vi "ClientDaemon.vi"(8 "error in (no error)":errorcluster, 10 "MessageReceiveQueue":refnum<queue>, 11 "mqtt.lvclass":refnum<class "MQTT Client.lvclass">) -> (0 "error out":errorcluster, 3 "mqtt.lvclass 2":refnum<class "MQTT Client.lvclass">)   [LabVIEW 2020, in "MQTT Client.lvclass"]
uses:
  MQTT Client.lvclass
  MqttMessage.ctl
  MQTT Client.lvclass/MQTT Client.ctl
  mqttTypedef/ReceivedData.ctl
  mqttTypedef/FixedHeaderResponse.ctl
  mqttTypedef/QosLevel.ctl
  mqttTypedef/MessageType.ctl
  mqttCmd/mqttCmdPublishAck/PublishAckMqttMsg.lvclass
  C:/Projects/Libraries/Gore SM 2020/mqtt-LabVIEW/src/class/mqtt/mqttCmd/BaseMqttMsg.lvclass
  mqttCmd/mqttCmdPublishReceived/PublishReceivedMqttMsg.lvclass
  mqttCmd/mqttCmdPublishComplete/PublishCompleteMqttMsg.lvclass
  mqttCmd/mqttCmdPingResponse/PingResponseMqttMsg.lvclass
  mqttCmd/BaseMqttMsg.lvclass
panel:
  out "rxCount":i32
  out "rxTelegram":u8[](array[numeric]) format="%02x"
  out "txError":errorcluster
  out "payloadError":errorcluster
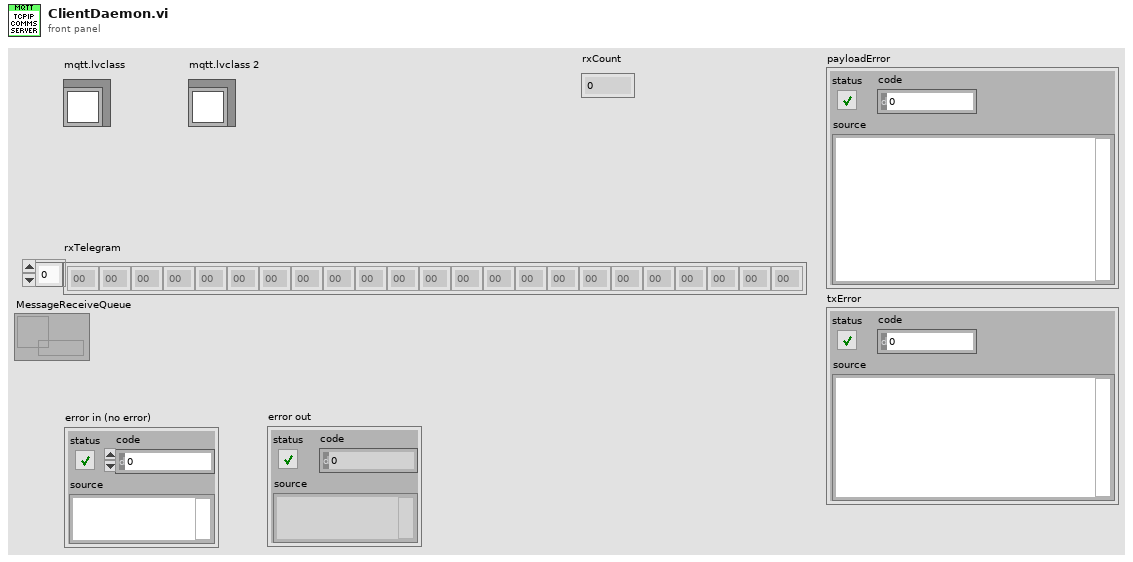
[diagram p1: front panel]
types:
  T1 = typedef "MQTT Client.lvclass/ReceivedData.ctl" = cluster{"fixedHdr":T2, "payload":u8[]}
  T2 = typedef "MQTT Client.lvclass/FixedHeaderResponse.ctl" = cluster{"retain":bool, "qos":T3, "duplicate":bool, "response":T4}
  T3 = typedef "MQTT Client.lvclass/QosLevel.ctl" = enum8{"At most once", "At least once", "Exactly once", "Reserved"}
  T4 = typedef "MQTT Client.lvclass/MessageType.ctl" = enum32{"Reserved", "CONNECT", "CONNACK", "PUBLISH", "PUBACK", "PUBREC", "PUBREL", "PUBCOMP", "SUBSCRIBE", "SUBACK", "UNSUBSCRIBE", "UNSUBACK", "PINGREQ", "PINGRESP", "DISCONNECT", "Reserved2"}
  T5 = cluster{"topic":string, "value":string, "messageID":u16}
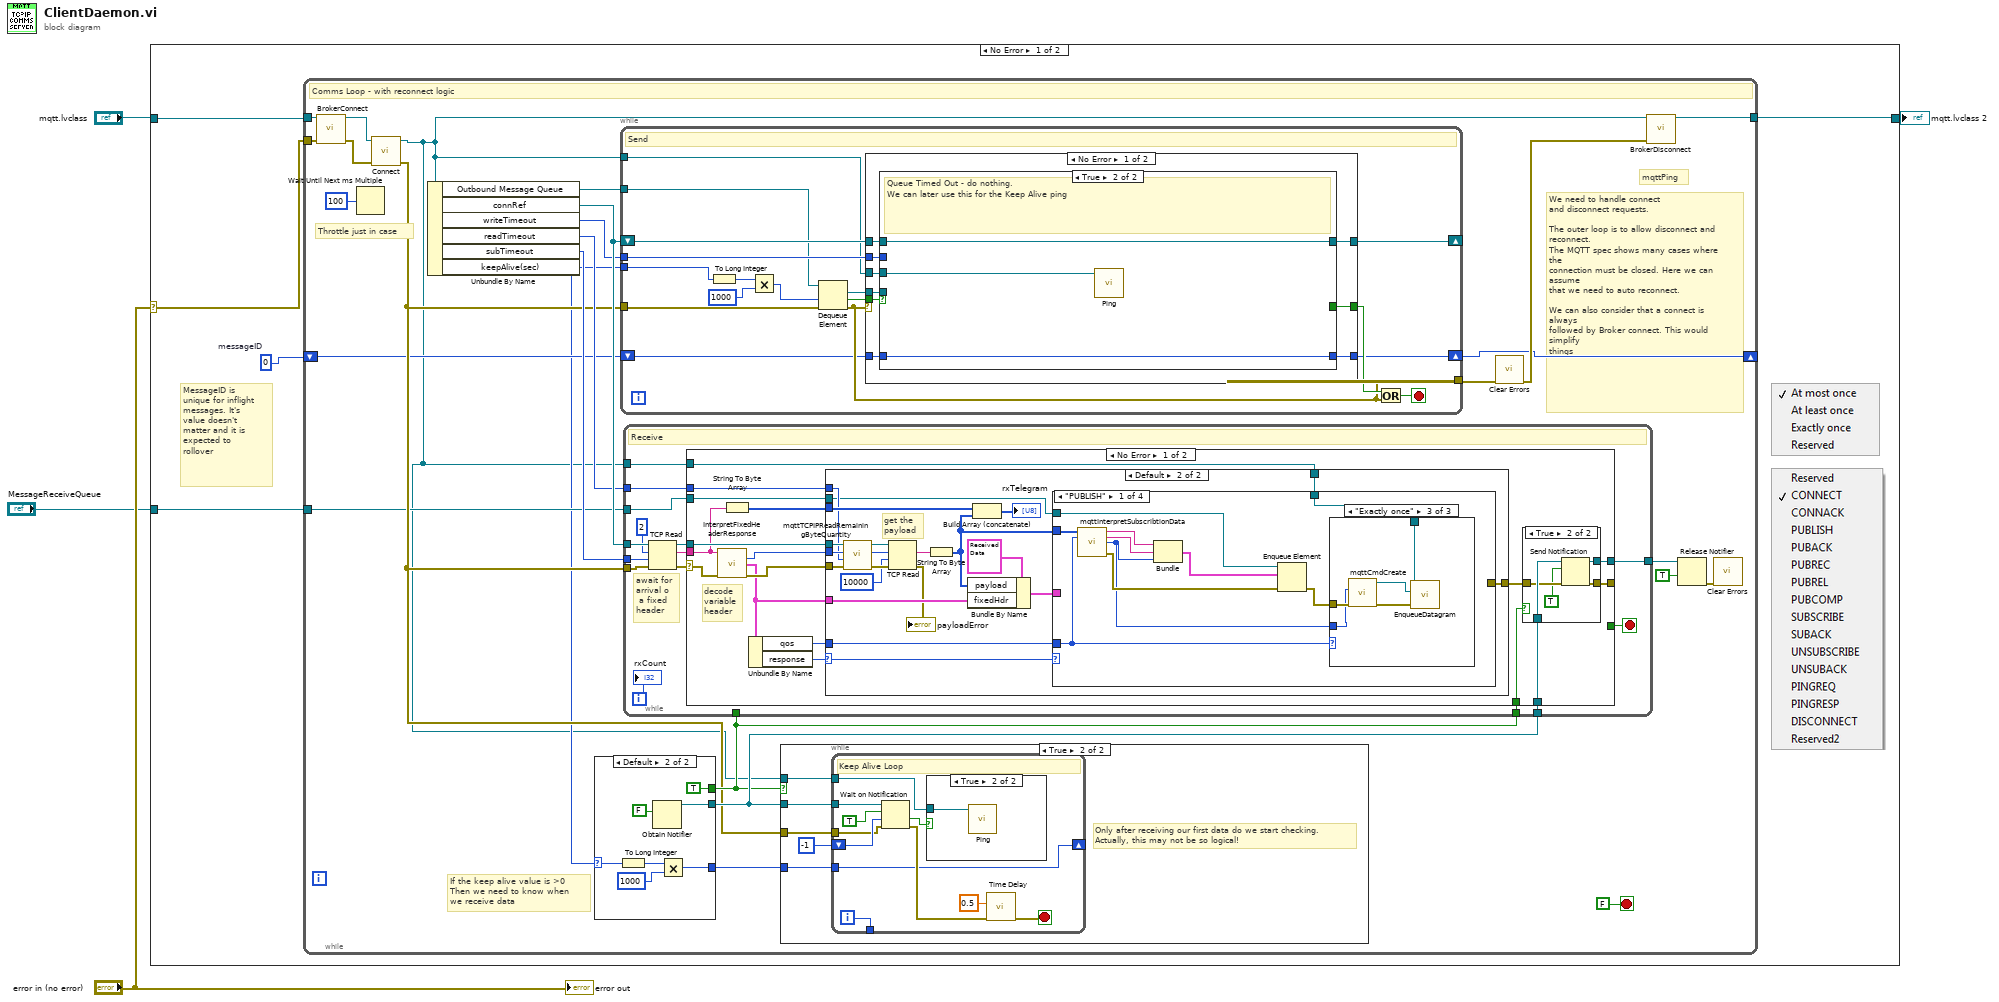
[diagram p0: block diagram]
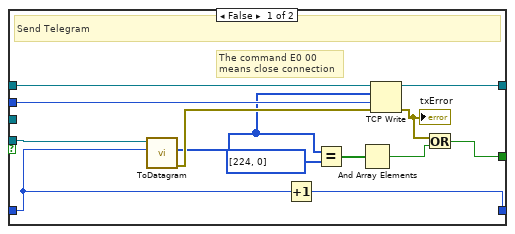
[diagram p5: hidden frame]
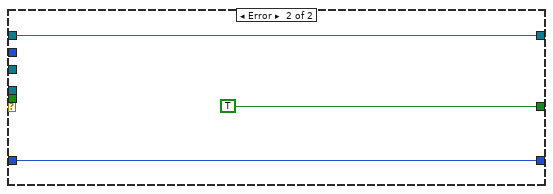
[diagram p6: hidden frame]
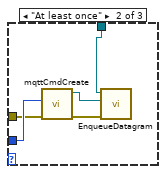
[diagram p10: hidden frame]
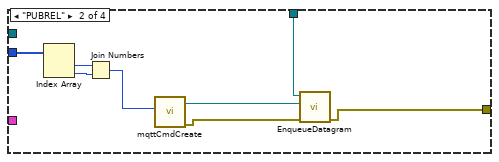
[diagram p11: hidden frame]
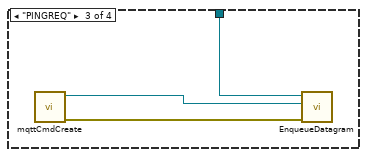
[diagram p12: hidden frame]
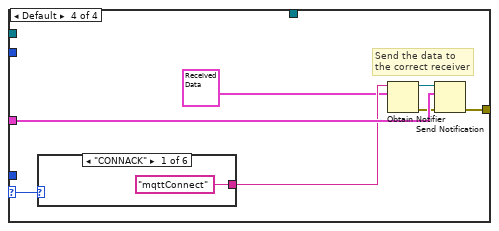
[diagram p13: hidden frame]
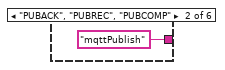
[diagram p14: hidden frame]
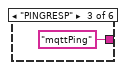
[diagram p15: hidden frame]
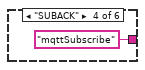
[diagram p16: hidden frame]
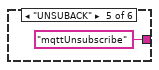
[diagram p17: hidden frame]
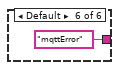
[diagram p18: hidden frame]
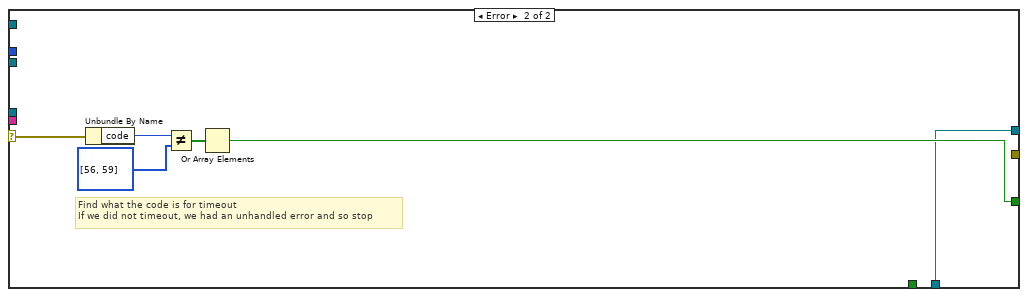
[diagram p19: hidden frame]
diagram:
  n1 = case shown="No Error" "error in (no error)" {
    selector: "error in (no error)" -> [w8 _]
    tunnel: "mqtt.lvclass" -> [w6 w213]
    tunnel: [w9 w213] -> w3
    tunnel: "MessageReceiveQueue" -> [w7 _]
    frame No Error {
      w5 = u16 0  # messageID
      # "MessageID is unique for inflight messages. It's value doesn't matter and it is expected to rollover"
      n2 = while {
        tunnel: w6 -> [w31]
        tunnel: [w29] -> w9
        tunnel: w8 -> [w30]
        tunnel: w7 -> [w17]
        shift-right: [w12] -> _
        shift-left: w5 -> [w13]
        stop <- FALSE stop-if-true
        # "We need to handle connect\nand disconnect requests.\n\nThe outer loop is to allow disconnect and reconnect.\nThe MQTT spec shows many cases where the\nconnection must be closed. Here we can assume\nthat we need to auto reconnect.\n\nWe can also consider that a connect is always\nfollowed by Broker connect. This would simplify\nthings"
        # "Throttle just in case"
        # "If the keep alive value is >0\nThen we need to know when\nwe receive data"
        # "mqttPing"
        # "Comms Loop - with reconnect logic"
        n3 = call "BrokerConnect.vi"("mqtt in"=w31, "error in (no error)"=w30) -> ("mqtt out"=w15:refnum<class "MQTT Client.lvclass">, "error out"=w19:errorcluster)  [unwired: 12 in]
        n4 = Wait Until Next ms Multiple(millisecond multiple=u32 100) -> ()  [unwired: 1 out]
        n5 = call "Connect.vi"("error in (no error)"=w19, "MQTT In"=w15) -> ("error out"=w18:errorcluster, "MQTT Out"=w10:refnum<class "MQTT Client.lvclass">)  [unwired: 8 in]
        n6 = Unbundle By Name(w10) -> ("Outbound Message Queue"=w14:refnum<queue>, "connRef"=w34:refnum<k5>, "writeTimeout"=w28:i32, "readTimeout"=w27:i32, "subTimeout"=w26:i32, "keepAlive(sec)"=w11:u16)
        n7 = case shown="Default" w11 {
          selector: w11 -> [_ w54]
          tunnel: [_ w59] -> w25
          tunnel: [_ w55] -> w21
          tunnel: [_ TRUE] -> w20
          frame ..0 {
          }
          frame Default {
            n8 = To Long Integer(number=w54) -> (32bit integer=w57:i32)
            n9 = Obtain Notifier(notification data type=FALSE) -> (notifier out=w59:refnum<notifier>)  [unwired: 3 in, 2 out]
            n10 = Multiply(x=w57, y=1000) -> (x*y=w55:i32)
          }
        }
        n11 = while {
          shift-right: [w74] -> _
          shift-left: w34 -> [w75]
          tunnel: [w70] -> w33
          tunnel: w28 -> [w69]
          tunnel: w18 -> [w68]
          tunnel: w14 -> [w67]
          shift-right: [w65] -> w12
          shift-left: w13 -> [w66]
          tunnel: w11 -> [w62]
          tunnel: w10 -> [w60]
          stop <- w73 stop-if-true
          # "Send"
          n12 = To Long Integer(number=w62) -> (32bit integer=w63:i32)
          n13 = Multiply(x=w63, y=1000) -> (x*y=w61:i32)
          n14 = Dequeue Element(queue=w67, timeout in ms (-1)=w61, error in (no error)=w68) -> (element=w71:refnum<class "BaseMqttMsg.lvclass">, timed out?=w76:bool, error out=w70:errorcluster)  [unwired: 1 out]
          n15 = case shown="No Error" w70 {
            tunnel: w76 -> [w85 _]
            tunnel: w71 -> [w84 _]
            tunnel: w75 -> [w83 w104]
            tunnel: [w82 w104] -> w74
            tunnel: [w81 TRUE] -> w72
            tunnel: w69 -> [w80 _]
            tunnel: w66 -> [w79 w102]
            tunnel: [w78 w102] -> w65
            tunnel: w60 -> [w77 _]
            frame No Error {
              n16 = case shown="True" w85 {
                tunnel: w84 -> [w90 _]
                tunnel: w83 -> [w98 w101]
                tunnel: [w97 w101] -> w82
                tunnel: [w91 _] -> w81
                tunnel: w80 -> [w94 _]
                tunnel: w79 -> [w87 w100]
                tunnel: [w86 w100] -> w78
                tunnel: w77 -> [_ w99]
                frame False {
                  # "The command E0 00\nmeans close connection"
                  # "Send Telegram"
                  n17 = call-dynamic "ToDatagram.vi"("messageID"=w87, "BaseMqttMsg in"=w90) -> ("error out"=w89:errorcluster, "Datagram"=w88:u8[])  [unwired: 7 in, 1 out]
                  n18 = Increment(x=w87) -> (x+1=w86:u16)
                  n19 = Equal?(x=w88, y=u8[] [224, 0] ("txTelegram 2")) -> (x = y?=w95:bool[])
                  n20 = And Array Elements(Boolean array=w95) -> (logical AND=w92:bool)
                  n21 = TCP Write(connection ID=w98, data in=w88, error in (no error)=w89, 9:w94) -> (connection ID out=w97:refnum<k5>, error out=w93:errorcluster)  [unwired: 1 out]
                  "txError" <- w93
                  n22 = Or(x=w93, y=w92) -> (x .or. y?=w91:bool)
                }
                frame True {
                  # "Queue Timed Out - do nothing.\nWe can later use this for the Keep Alive ping"
                  n23 = call "Ping.vi"("mqtt in"=w99) -> ()  [unwired: 9 in, 2 out]
                }
              }
            }
            frame Error {
            }
          }
          n24 = Or(x=w72, y=w70) -> (x .or. y?=w73:bool)
        }
        n25 = while {
          tunnel: w34 -> [w119]
          tunnel: w27 -> [w112]
          tunnel: w26 -> [w111]
          tunnel: w25 -> [w110]
          tunnel: [w109] -> w24
          tunnel: w20 -> [w108]
          tunnel: w20 -> [_]
          tunnel: w18 -> [w107]
          tunnel: w17 -> [w106]
          tunnel: w10 -> [w105]
          i -> [w113]
          stop <- w114 stop-if-true
          # "await for\narrival o\n a fixed\nheader"
          # "Receive"
          n26 = TCP Read(connection ID=w119, bytes to read=2, error in (no error)=w107, 9:w111) -> (connection ID out=w118:refnum<k5>, data out=w115:string, error out=w117:errorcluster)  [unwired: 1 in]
          n27 = case shown="No Error" w117 {
            selector: w117 -> [w134 w212]
            tunnel: w118 -> [w135 _]
            tunnel: w115 -> [w130 _]
            tunnel: [_ w208] -> w114
            tunnel: w112 -> [w127 _]
            tunnel: w110 -> [w126 w207]
            tunnel: [w124 w207] -> w109
            tunnel: [w123 _] -> _
            tunnel: w108 -> [w122 _]
            tunnel: w106 -> [w121 _]
            tunnel: w105 -> [w120 _]
            frame No Error {
              # "decode\nvariable\nheader"
              n28 = call "InterpretFixedHeaderResponse.vi"("data in"=w130, "error in (no error)"=w134) -> ("remainingLengthByte1"=w136:u8, "output cluster"=w132:T2, "error out"=w133:errorcluster)  [unwired: 11 in]
              n29 = String To Byte Array(string=w130) -> (unsigned byte array=w129:u8[])
              n30 = Unbundle By Name(w132) -> ("qos"=w128:T3, "response"=w131:T4)
              n31 = case shown="Default" w131 {
                selector: w131 -> [_ w152]
                tunnel: w136 -> [_ w162]
                tunnel: w135 -> [_ w161]
                tunnel: w133 -> [_ w154]
                tunnel: w132 -> [_ w153]
                tunnel: w129 -> [_ w149]
                tunnel: w128 -> [_ w148]
                tunnel: w127 -> [_ w145]
                tunnel: [_ w144] -> w125
                tunnel: w121 -> [_ w143]
                tunnel: w120 -> [_ w142]
                frame "CONNECT", "SUBSCRIBE" {
                  # "The client should not receive these commands.\nI had some problems with these commands being received\nand it appears this was a broker issue. However, to ignore\nmessages that we should not receive is no bad thing."
                }
                frame Default {
                  # "get the\npayload"
                  n32 = call "mqttTCPIPReadRemainingByteQuantity.vi"("error in (no error)"=w154, "readTimeout ms (2000)"=w145, "remainingLengthByte1"=w162, "connRef in"=w161) -> ("error out"=w159:errorcluster, "remainingLength"=w158:i32, "connRef out"=w160:refnum<k5>)  [unwired: 5 in]
                  n33 = TCP Read(connection ID=w160, bytes to read=w158, error in (no error)=w159, 9:10000 ("timeout ms (25000)")) -> (data out=w156:string, error out=→"payloadError":errorcluster)  [unwired: 1 in, 1 out]
                  n34 = String To Byte Array(string=w156) -> (unsigned byte array=w146:u8[])
                  n35 = Bundle By Name(cluster=T1 {"fixedHdr"={"retain"=FALSE, "qos"=enum."At most once", "duplicate"=FALSE, "response"=enum."Reserved"}, "payload"=[]} ("output cluster"), "payload"=w146, "fixedHdr"=w153) -> (w150:T1)
                  n36 = Build Array (concatenate)(w149, w146) -> (→"rxTelegram":u8[])
                  n37 = case shown="\"PUBLISH\"" w152 {
                    selector: w152 -> [_ _ _ w200]
                    tunnel: w150 -> [_ _ _ w199]
                    tunnel: w148 -> [w171 _ _ _]
                    tunnel: w146 -> [w172 w190 _ _]
                    tunnel: [_ w183 _ w194] -> w144
                    tunnel: w143 -> [w170 _ _ _]
                    tunnel: w142 -> [w167 w185 w193 _]
                    frame "PUBLISH" {
                      n38 = call "mqttInterpretSubscribtionData.vi"("rxTelegram in"=w172, "qos"=w171) -> ("topic"=w166:string, "value"=w165:string, "messageID"=w164:u16, "error out"=w168:errorcluster)  [unwired: 10 in]
                      n39 = Bundle("topic"=w166, "value"=w165, "messageID"=w164) -> (w163:T5)  [unwired: 1 in]
                      n40 = Enqueue Element(queue=w170, element=w163, error in (no error)=w168) -> (error out=w169:errorcluster)  [unwired: 1 in, 2 out]
                      n41 = case shown="\"Exactly once\"" w171 {
                        tunnel: w169 -> [_ w176 w182]
                        tunnel: w164 -> [_ w177 w181]
                        tunnel: w167 -> [_ w174 w178]
                        frame Default {
                        }
                        frame "At least once" {
                          n42 = call "mqttCmdCreate.vi"("error in (no error)"=w176, "messageID"=w177) -> ("error out"=w173:errorcluster, "mqttCmdPublishAck out"=w175:refnum<class "PublishAckMqttMsg.lvclass">)  [unwired: 8 in]
                          n43 = call "EnqueueDatagram.vi"("error in (no error)"=w173, "mqttCmd"=w175, "mqtt in"=w174) -> ()  [unwired: 7 in, 2 out]
                        }
                        frame "Exactly once" {
                          n44 = call "mqttCmdCreate.vi"("error in (no error)"=w182, "messageID"=w181) -> ("error out"=w180:errorcluster, "mqttCmdPublishReceived out"=w179:refnum<class "PublishReceivedMqttMsg.lvclass">)  [unwired: 8 in]
                          n45 = call "EnqueueDatagram.vi"("error in (no error)"=w180, "mqttCmd"=w179, "mqtt in"=w178) -> ()  [unwired: 7 in, 2 out]
                        }
                      }
                    }
                    frame "PUBREL" {
                      n46 = Index Array(array=w190) -> (element #1=w189:u8, element #2=w188:u8)  [unwired: 2 in]
                      n47 = Join Numbers(hi=w189, lo=w188) -> ((hi.lo)=w187:u16)
                      n48 = call "mqttCmdCreate.vi"("messageID"=w187) -> ("error out"=w184:errorcluster, "mqttCmdPublishComplete out"=w186:refnum<class "PublishCompleteMqttMsg.lvclass">)  [unwired: 9 in]
                      n49 = call "EnqueueDatagram.vi"("error in (no error)"=w184, "mqttCmd"=w186, "mqtt in"=w185) -> ("error out"=w183:errorcluster)  [unwired: 7 in, 1 out]
                    }
                    frame "PINGREQ" {
                      n50 = call "mqttCmdCreate.vi"() -> ("error out"=w191:errorcluster, "mqttCmdPingResponse out"=w192:refnum<class "PingResponseMqttMsg.lvclass">)  [unwired: 10 in]
                      n51 = call "EnqueueDatagram.vi"("error in (no error)"=w191, "mqttCmd"=w192, "mqtt in"=w193) -> ()  [unwired: 7 in, 2 out]
                    }
                    frame Default {
                      # "Send the data to\nthe correct receiver"
                      n52 = case shown="\"CONNACK\"" w200 {
                        tunnel: ["mqttConnect" ("name (unnamed)") "mqttPublish" ("name (unnamed)") "mqttPing" ("name (unnamed)") "mqttSubscribe" ("name (unnamed)") "mqttUnsubscribe" ("name (unnamed)") "mqttError" ("name (unnamed)")] -> w198
                        frame "CONNACK" {
                        }
                        frame "PUBACK", "PUBREC", "PUBCOMP" {
                        }
                        frame "PINGRESP" {
                        }
                        frame "SUBACK" {
                        }
                        frame "UNSUBACK" {
                        }
                        frame Default {
                        }
                      }
                      n53 = Obtain Notifier(name (unnamed)=w198, notification data type=T1 {"fixedHdr"={"retain"=FALSE, "qos"=enum."At most once", "duplicate"=FALSE, "response"=enum."Reserved"}, "payload"=[]} ("output cluster")) -> (notifier out=w197:refnum<notifier>, error out=w195:errorcluster)  [unwired: 2 in, 1 out]
                      n54 = Send Notification(notification=w199, notifier=w197, error in (no error)=w195) -> (error out=w194:errorcluster)  [unwired: 1 out]
                    }
                  }
                }
              }
              n55 = case shown="True" w122 {
                tunnel: w126 -> [_ w141]
                tunnel: w125 -> [_ w140]
                tunnel: [_ w138] -> w124
                tunnel: [_ w137] -> w123
                frame False {
                }
                frame True {
                  n56 = Send Notification(notification=TRUE, notifier=w141, error in (no error)=w140) -> (notifier out=w138:refnum<notifier>, error out=w137:errorcluster)
                }
              }
            }
            frame Error {
              # "Find what the code is for timeout\nIf we did not timeout, we had an unhandled error and so stop"
              n57 = Unbundle By Name(w212) -> ("code"=w211:i32)
              n58 = Not Equal?(x=w211, y=i32[] [56, 59]) -> (x != y?=w209:bool[])
              n59 = Or Array Elements(Boolean array=w209) -> (logical OR=w208:bool)
            }
          }
          "rxCount" <- w113
        }
        n60 = case shown="True" w20 {
          tunnel: w25 -> [_ w40]
          tunnel: w21 -> [_ w39]
          tunnel: w18 -> [_ w37]
          tunnel: w10 -> [_ w36]
          frame False {
          }
          frame True {
            # "Only after receiving our first data do we start checking.\nActually, this may not be so logical!"
            n61 = while {
              tunnel: w40 -> [w51]
              tunnel: [w47] -> _
              shift-right: [w44] -> _
              shift-left: -1 -> [w50]
              tunnel: w39 -> [w44]
              tunnel: w37 -> [w43]
              tunnel: w36 -> [w42]
              i -> [w47]
              stop <- w48 stop-if-true
              # "Keep Alive Loop"
              n62 = Wait on Notification(notifier=w51, ignore previous (F)=TRUE, timeout in ms (-1)=w50, error in (no error)=w43) -> (timed out?=w41:bool, error out=w45:errorcluster)  [unwired: 2 out]
              n63 = case shown="True" w41 {
                tunnel: w42 -> [_ w52]
                frame False {
                }
                frame True {
                  n64 = call "Ping.vi"("mqtt in"=w52) -> ()  [unwired: 9 in, 2 out]
                }
              }
              n65 = call "Time Delay"("error in (no error)"=w45, "Delay Time (s)"=0.5) -> ("error out"=w48:errorcluster)  [unwired: 9 in]
            }
          }
        }
        n66 = call <vilib>:"Clear Errors.vi"("error in (no error)"=w33) -> ("error out"=w32:errorcluster)  [unwired: 5 in, 1 out]
        n67 = call "BrokerDisconnect.vi"("mqtt in"=w10, "error in (no error)"=w32) -> ("mqtt out"=w29:refnum<class "MQTT Client.lvclass">)  [unwired: 12 in, 1 out]
        n68 = Release Notifier(notifier=w24, force destroy? (F)=TRUE) -> (error out=w22:errorcluster)  [unwired: 1 in, 2 out]
        n69 = call <vilib>:"Clear Errors.vi"("error in (no error)"=w22) -> ()  [unwired: 5 in, 2 out]
      }
    }
    frame Error {
    }
  }
  "mqtt.lvclass 2" <- w3
  "error out" <- "error in (no error)"
